vi "32xI16 Packer to 24xI16 Packer_debug.vi"(8 "Input Data Valid":bool, 11 "Input 32xI16 Array":i16[](array[numeric])=[0, -16, -32, -48, -64, -80, -96, -112, -128, -144, -160, -176, -192, -208, -224, -240, -256, -272, -288, -304, -320, -336, -352, -368, -384, -400, -416, -432, -448, -464, -480, -496] format="%016b") -> (0 "Output Valid":bool, 3 "Output Data":i16[](array[numeric])=[255, -1, -1, -1, -1, -1, -1, -1, -1793, -2050, -2306, -2562, -2818, -3074, -3330, -3586, 4072, -25, -4122, -8219, -12316, -16413, -20510, -24607])   [LabVIEW 2012]
panel:
  out "Set 3":i16[](array[numeric])=[4072, -25, -4122, -8219, -12316, -16413, -20510, -24607] format="%016b"
  out "Set 2":i16[](array[numeric])=[-1793, -2050, -2306, -2562, -2818, -3074, -3330, -3586] format="%016b"
  out "Set 1":i16[](array[numeric])=[255, -1, -1, -1, -1, -1, -1, -1] format="%016b"
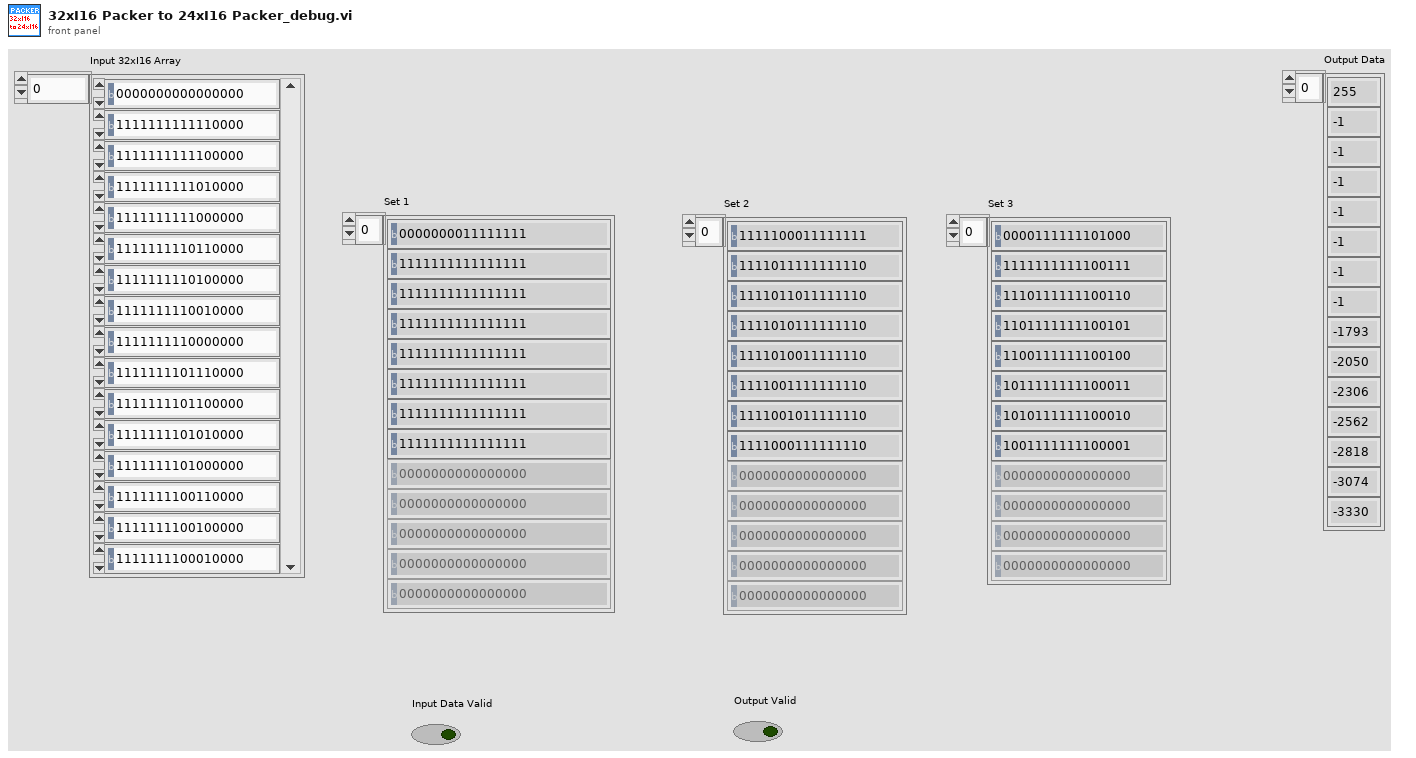
[diagram p1: front panel]
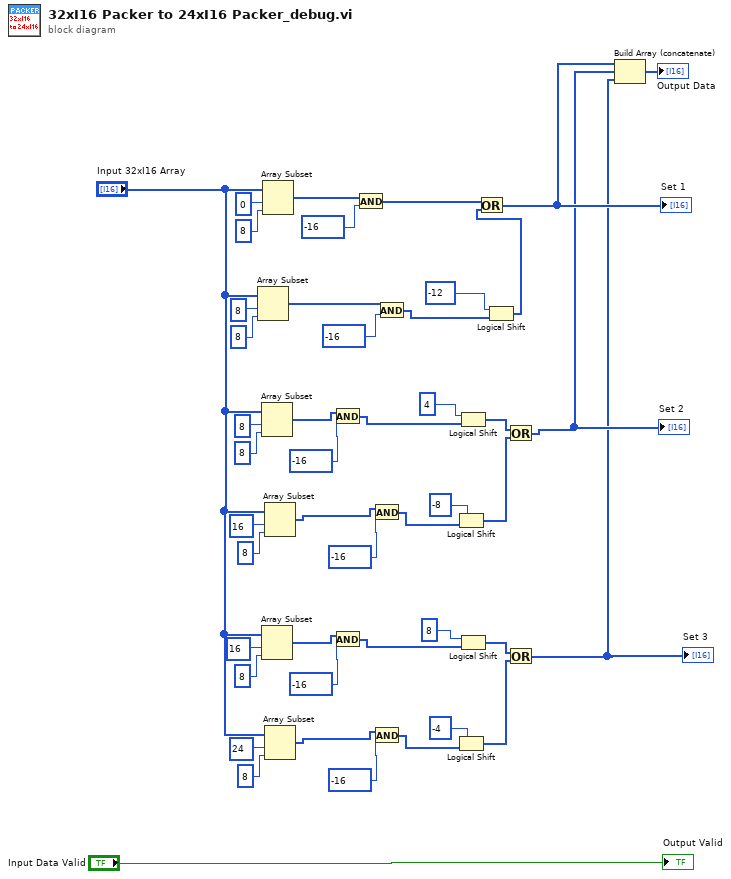
[diagram p0: block diagram]
diagram:
  n1 = Array Subset(array="Input 32xI16 Array", index=8, length=8 ("index")) -> (w7:i16[])
  n2 = Array Subset(array="Input 32xI16 Array", index=8, length=8 ("index")) -> (w29:i16[])
  n3 = Array Subset(array="Input 32xI16 Array", index=16, length=8 ("index")) -> (w18:i16[])
  n4 = Array Subset(array="Input 32xI16 Array", index=0, length=8 ("index")) -> (w39:i16[])
  n5 = Array Subset(array="Input 32xI16 Array", index=16, length=8 ("index")) -> (w25:i16[])
  n6 = Array Subset(array="Input 32xI16 Array", index=24, length=8 ("index")) -> (w22:i16[])
  n7 = And(x=w29, y=i16 -16) -> (x .and. y?=w27:i16[])
  n8 = And(x=w18, y=i16 -16) -> (x .and. y?=w20:i16[])
  n9 = And(x=w39, y=i16 -16) -> (x .and. y?=w44:i16[])
  n10 = And(x=w25, y=i16 -16) -> (x .and. y?=w24:i16[])
  n11 = And(x=w22, y=i16 -16) -> (x .and. y?=w23:i16[])
  n12 = And(x=w7, y=i16 -16) -> (x .and. y?=w6:i16[])
  n13 = Logical Shift(y=i16 -8, x=w24) -> (x << y=w31:i16[])
  n14 = Logical Shift(y=i16 -4, x=w23) -> (x << y=w17:i16[])
  n15 = Logical Shift(y=i16 4, x=w27) -> (x << y=w32:i16[])
  n16 = Logical Shift(y=i16 8, x=w20) -> (x << y=w16:i16[])
  n17 = Logical Shift(y=i16 -12, x=w6) -> (x << y=w33:i16[])
  n18 = Or(x=w44, y=w33) -> (x .or. y?=w5:i16[])
  "Set 1" <- w5
  n19 = Or(x=w32, y=w31) -> (x .or. y?=w4:i16[])
  "Set 2" <- w4
  n20 = Or(x=w16, y=w17) -> (x .or. y?=w3:i16[])
  "Set 3" <- w3
  n21 = Build Array (concatenate)(w5, w4, w3) -> (→"Output Data":i16[])
  "Output Valid" <- "Input Data Valid"
